vi "Clear Processes.vi"(8 "error in (no error)":errorcluster, 11 "Application In":refnum<class "Application.lvclass">) -> (0 "error out":errorcluster, 3 "Application Out":refnum<class "Application.lvclass">)   [LabVIEW 2020, in "Application.lvclass"]
uses:
  Application.lvclass
  Application.lvclass/Application.ctl
  Process/Process.lvclass
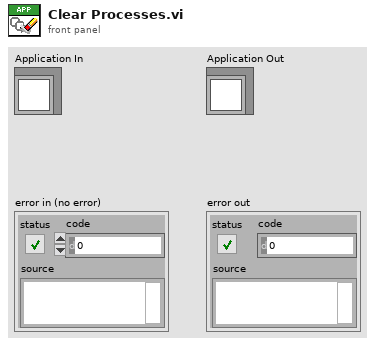
[diagram p1: front panel]
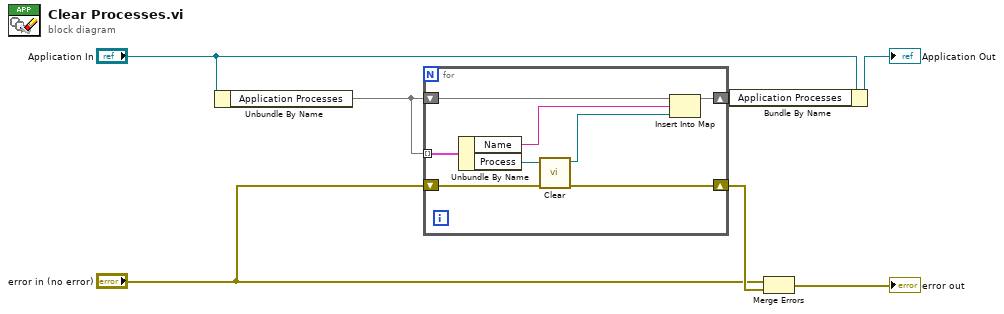
[diagram p0: block diagram]
diagram:
  n1 = Unbundle By Name("Application In") -> ("Application Processes"=w4:map{string, refnum<class "Process.lvclass">})
  n2 = for {
    shift-right: [w15] -> w6
    shift-left: "error in (no error)" -> [w14]
    tunnel: w4 -> [w13] mode=indexing
    shift-right: [w9] -> w2
    shift-left: w4 -> [w10]
    n3 = Unbundle By Name(w13) -> ("Name"=w8:string, "Process"=w11:refnum<class "Process.lvclass">)
    n4 = call-dynamic "Clear.vi"("error in (no error)"=w14, "Process In"=w11) -> ("error out"=w15:errorcluster, "Process Out"=w12:refnum<class "Process.lvclass">)  [unwired: 8 in]
    n5 = Insert Into Map(map in=w10, key=w8, value=w12) -> (map out=w9:map{string, refnum<class "Process.lvclass">})  [unwired: 2 out]
  }
  n6 = Bundle By Name(cluster="Application In", "Application Processes"=w2) -> (→"Application Out":refnum<class "Application.lvclass">)
  n7 = Merge Errors("error in (no error)", w6) -> (→"error out":errorcluster)
